vi "Create myVTOL.vi"(8 "error in (no error)":errorcluster, 10 "device name (myDAQ1)":tag="myDAQ1") -> (0 "error out":errorcluster, 2 "connection failed?":bool, 3 "task array out":refnum<k21>[](array[refnum]))   [LabVIEW 2013]
doc: "Creates an array of 2 DAQmx tasks used in myVTOL\nUse the <b> device name</b> input to select the myDAQ you want to use. \n\nAnalog Input 0 Hall Effect Voltage\nAnalog Output 0 Fan Motor Drive"
uses:
  <vilib>/DAQmx/create/channels.llb/DAQmx Create Channel (AI-Voltage-Basic).vi
  <vilib>/DAQmx/create/channels.llb/DAQmx Create Channel (AO-Voltage-Basic).vi
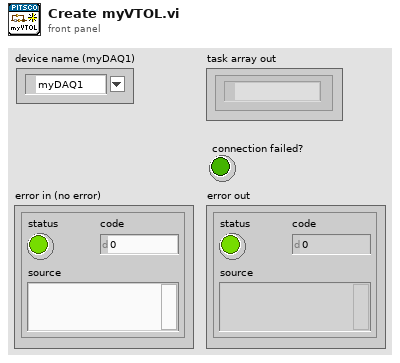
[diagram p1: front panel]
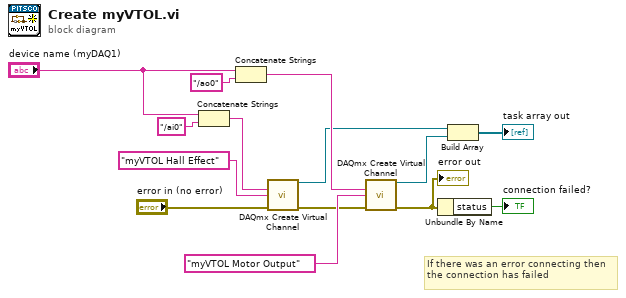
[diagram p0: block diagram]
diagram:
  # "If there was an error connecting then the connection has failed"
  n1 = Concatenate Strings("device name (myDAQ1)", "/ai0" ("string")) -> (w11:string)
  n2 = Concatenate Strings("device name (myDAQ1)", "/ao0" ("string")) -> (w10:string)
  n3 = call-poly <vilib>:"DAQmx Create Virtual Channel.vi"("physical channels"=w11, "name to assign"="myVTOL Hall Effect" ("Descr (myDAQ AI)"), "error in"="error in (no error)") -> ("task out"=w1:refnum<k21>, "error out"=w2:errorcluster)  [unwired: 11 in]
  n4 = call-poly <vilib>:"DAQmx Create Virtual Channel.vi"("physical channels"=w10, "name to assign"="myVTOL Motor Output", "error in"=w2) -> ("task out"=w8:refnum<k21>, "error out"=w3:errorcluster)  [unwired: 11 in]
  "error out" <- w3
  n5 = Unbundle By Name(w3) -> ("status"=→"connection failed?":bool)
  n6 = Build Array(w1, w8) -> (→"task array out":refnum<k21>[])
